vi "Load config.vi"(8 "error in (no error)":errorcluster) -> (0 "error out":errorcluster, 2 "Camera config":T1, 3 "Arduino config":T3)   [LabVIEW 2020]
uses:
  controls/Arduino config -- cluster.ctl
  controls/Camera config parameters -- cluster.ctl
  <vilib>/userdefined/High Color/IMAQdx.ctl
  <vilib>/Utility/config.llb/Read Key (String).vi
  <vilib>/Utility/config.llb/Read Key (U32).vi
  <vilib>/Utility/config.llb/NI_LVConfig.lvlib
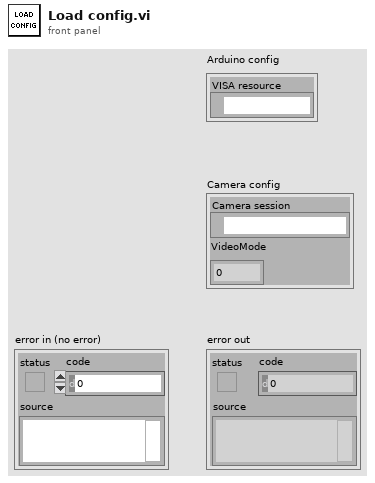
[diagram p1: front panel]
types:
  T1 = typedef "Camera config parameters -- cluster.ctl" = cluster{"Camera session":T2, "VideoMode":u32}
  T2 = typedef "IMAQdx.ctl" = refnum<k21>
  T3 = typedef "Arduino config -- cluster.ctl" = cluster{"VISA resource":refnum<visa-resource-name>}
  T4 = typedef "NI_LVConfig.lvlib/Config Data RefNum.ctl" = refnum<k1>
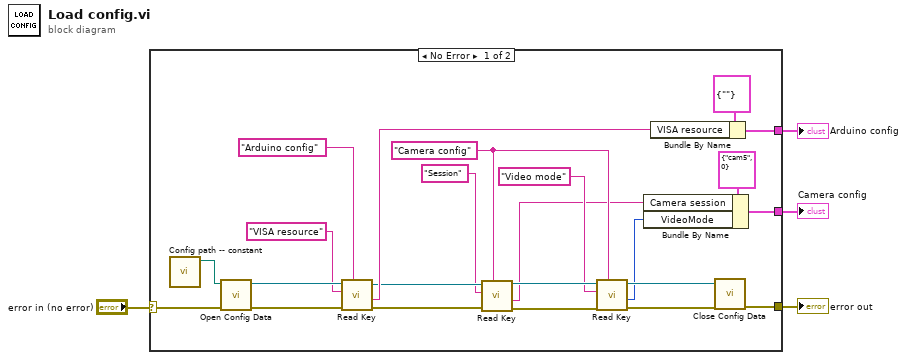
[diagram p0: block diagram]
diagram:
  n1 = case shown="No Error" "error in (no error)" {
    selector: "error in (no error)" -> [w26 w28]
    tunnel: [w25 w28] -> w3
    tunnel: [w18 _] -> w2
    tunnel: [w16 _] -> w1
    frame No Error {
      w11 = "Camera config" ("section")
      n2 = call "Config path -- constant.vi"() -> ("appended path"=w27:path)  [unwired: 11 in]
      n3 = call <vilib>:"Open Config Data.vi"("error in (no error)"=w26, "configuration file path"=w27) -> ("error out"=w24:errorcluster, "refnum"=w22:T4)  [unwired: 7 in, 1 out]
      n4 = call-poly <vilib>:"Read Key.vi"("section"="Arduino config", "error in (no error)"=w24, "key"="VISA resource", "refnum"=w22) -> ("error out"=w15:errorcluster, "value"=w19:string, "refnum out"=w14:T4)  [unwired: 4 in, 1 out]
      n5 = call-poly <vilib>:"Read Key.vi"("section"=w11, "error in (no error)"=w15, "key"="Session", "refnum"=w14) -> ("error out"=w13:errorcluster, "value"=w6:string, "refnum out"=w12:T4)  [unwired: 4 in, 1 out]
      n6 = call-poly <vilib>:"Read Key.vi"("section"=w11, "error in (no error)"=w13, "key"="Video mode", "refnum"=w12) -> ("error out"=w8:errorcluster, "value"=w5:u32, "refnum out"=w7:T4)  [unwired: 4 in, 1 out]
      n7 = Bundle By Name(cluster=T1 {"Camera session"="cam5", "VideoMode"=0} ("Camera config"), "Camera session"=w6, "VideoMode"=w5) -> (w16:T1)
      n8 = Bundle By Name(cluster=T3 {"VISA resource"=""} ("Arduino config"), "VISA resource"=w19) -> (w18:T3)
      n9 = call <vilib>:"Close Config Data.vi"("error in (no error)"=w8, "refnum"=w7) -> ("error out"=w25:errorcluster)  [unwired: 8 in, 1 out]
    }
    frame Error {
    }
  }
  "error out" <- w3
  "Arduino config" <- w2
  "Camera config" <- w1
